vi "processAndUpdateAI.vi"(8 "error in (no error)":errorcluster, 10 "data in":waveform(dbl)[](array[waveform]), 11 "Channels":refnum<k21>[](array[refnum])) -> (0 "error out":errorcluster)   [LabVIEW 2011, in "DaqPad_NI6009.lvclass"]
uses:
  DaqPad_NI6009.lvclass
  NI_AALBase.lvlib
panel:
  out "concatenated string":string
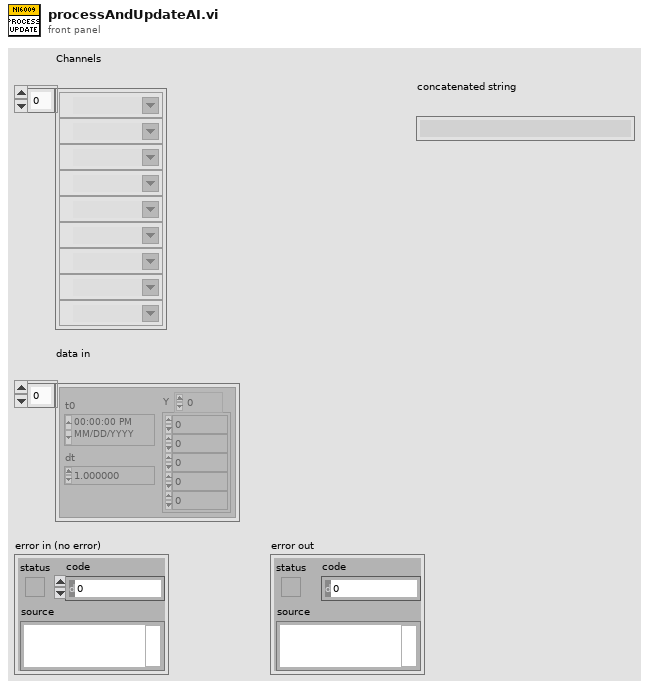
[diagram p1: front panel]
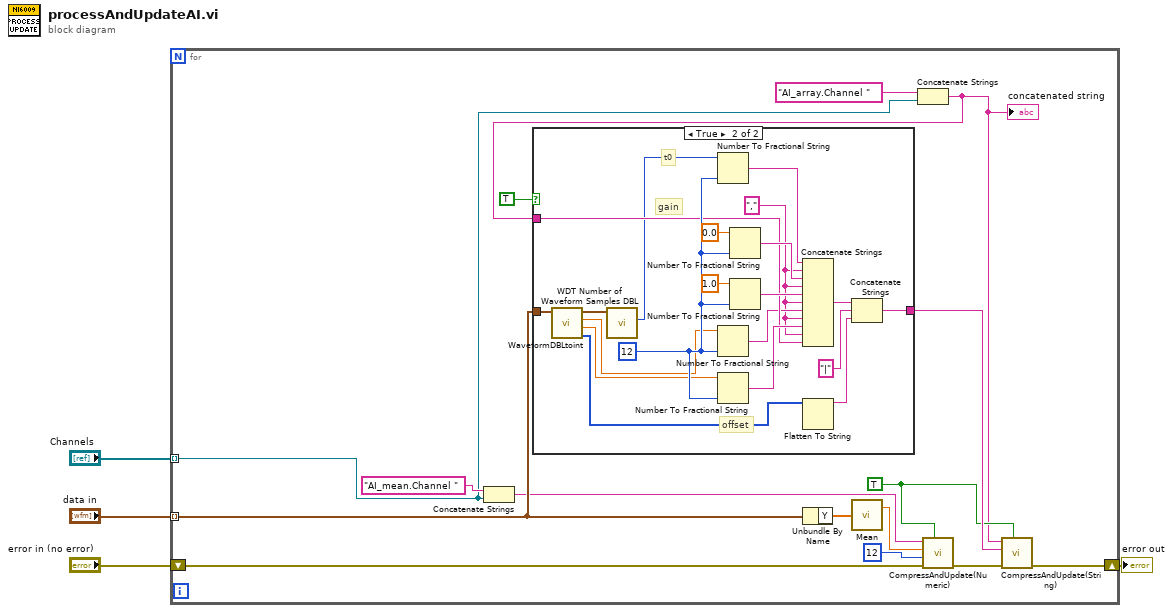
[diagram p0: block diagram]
diagram:
  n1 = for {
    tunnel: "data in" -> [w13] mode=indexing
    tunnel: "Channels" -> [w6] mode=indexing
    shift-right: [w15] -> w3
    shift-left: "error in (no error)" -> [w18]
    w8 = TRUE ("force CVT update (false)")
    n2 = Concatenate Strings("AI_mean.Channel " ("string"), w6) -> (w12:string)
    n3 = Unbundle By Name(w13) -> ("Y"=w14:dbl[])
    n4 = call "Mean.vi"("X"=w14) -> ("mean"=w9:dbl)  [unwired: 1 out]
    n5 = Concatenate Strings("AI_array.Channel " ("string"), w6) -> (w5:string)
    "concatenated string" <- w5
    n6 = case shown="True" TRUE {
      tunnel: [_ w31] -> w11
      tunnel: w5 -> [_ w30]
      tunnel: w13 -> [_ w21]
      frame False {
      }
      frame True {
        w35 = i16 12 ("precision (6)")
        w28 = "," ("string")
        # "gain"
        # "offset"
        # "t0"
        n7 = call "WaveformDBLtoint.vi"("Waveform"=w21) -> ("32bit integer"=w25:i16[], "scale"=w23:dbl, "offset"=w24:dbl, "waveform out"=w20:waveform(dbl))  [unwired: 7 in]
        n8 = call "WDT Number of Waveform Samples DBL.vi"("waveform in"=w20) -> ("number of samples"=w27:i32)  [unwired: 8 in, 2 out]
        n9 = Number To Fractional String(number=w27, precision (6)=w35) -> (F-format string=w39:string)  [unwired: 2 in]
        n10 = Number To Fractional String(number=w24, precision (6)=w35) -> (F-format string=w29:string)  [unwired: 2 in]
        n11 = Number To Fractional String(number=w23, precision (6)=w35) -> (F-format string=w36:string)  [unwired: 2 in]
        n12 = Number To Fractional String(number=0.0, precision (6)=w35) -> (F-format string=w38:string)  [unwired: 2 in]
        n13 = Number To Fractional String(number=1.0, precision (6)=w35) -> (F-format string=w37:string)  [unwired: 2 in]
        n14 = Concatenate Strings(w39, w28, w38, w28, w37, w28, w29, w28, w36, w28, w30) -> (w34:string)
        n15 = Flatten To String(anything=w25) -> (data string=w32:string)  [unwired: 3 in, 2 out]
        n16 = Concatenate Strings(w34, "|" ("string"), w32) -> (w31:string)
      }
    }
    n17 = call "CompressAndUpdate(Numeric).vi"("force CVT update (false)"=w8, "error in"=w18, "precision (6)"=i16 12, "Numeric"=w9, "command or variable name"=w12) -> ("error out"=w17:errorcluster)  [unwired: 6 in]
    n18 = call "CompressAndUpdate(String).vi"("force CVT update (false)"=w8, "error in"=w17, "String"=w11, "command or variable name"=w5) -> ("error out"=w15:errorcluster)  [unwired: 7 in]
  }
  "error out" <- w3
